vi "Do Request.vi"(7 "Controller Inputs":T2, 8 "error in (no error)":errorcluster, 11 "TestCSRFController in":refnum<class "TestCSRFController.lvclass">) -> (0 "error out":errorcluster, 5 "Controller Outputs":T1)   [LabVIEW 2020, in "TestCSRFController.lvclass"]
uses:
  TestCSRFController.lvclass
  HTTP Server/Controller Inputs.ctl
  HTTP Server/Arguments/Arguments.lvclass
  <vilib>/IlluminatedG/IG HTTP Utils/HTTP Utils/Request/Request.lvclass
  HTTP Server/Session/Session.lvclass
  HTTP Server/Controller Outputs.ctl
  <vilib>/IlluminatedG/IG HTTP Utils/HTTP Utils/Response/Response.lvclass
  TestCSRFController.lvclass/TestCSRFController.ctl
  <vilib>/IlluminatedG/IG HTTP Utils/HTTP Utils/FormField/FormField.lvclass
  HTTP Server/HTTP Server.lvlib
  <vilib>/IlluminatedG/lv-stream/URI/URI.lvclass
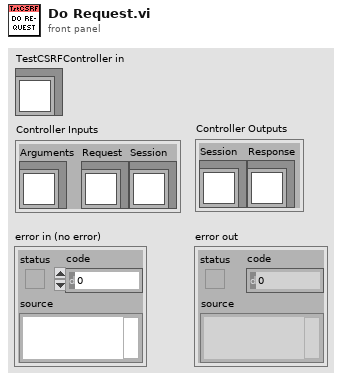
[diagram p1: front panel]
types:
  T1 = typedef "HTTP Server.lvlib/Controller Outputs.ctl" = cluster{"Session":refnum<class "Session.lvclass">, "Response":refnum<class "Response.lvclass">}
  T2 = typedef "HTTP Server.lvlib/Controller Inputs.ctl" = cluster{"Arguments":refnum<class "Arguments.lvclass">, "Request":refnum<class "Request.lvclass">, "Session":refnum<class "Session.lvclass">}
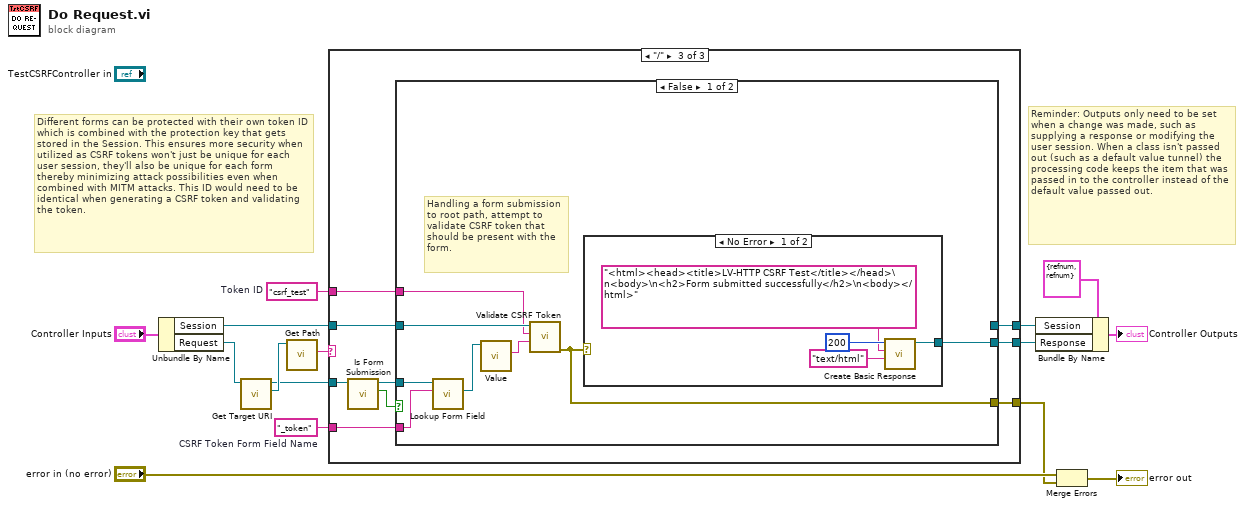
[diagram p0: block diagram]
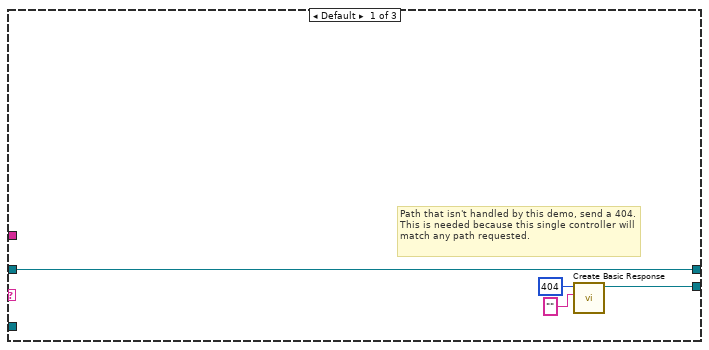
[diagram p2: hidden frame]
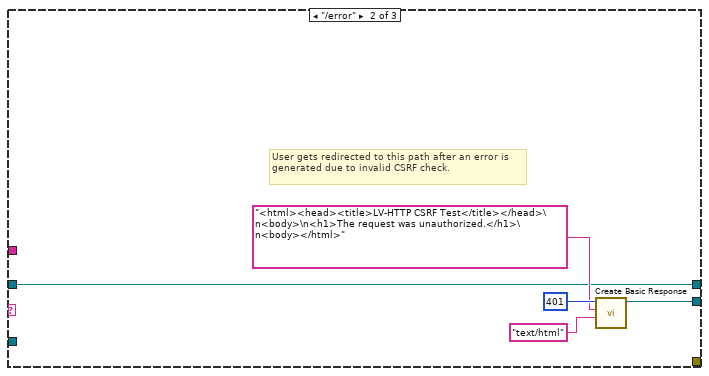
[diagram p3: hidden frame]
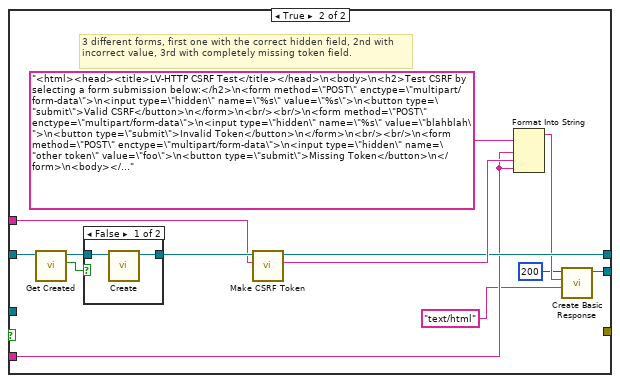
[diagram p5: hidden frame]
diagram:
  w11 = "_token"  # CSRF Token Form Field Name
  w12 = "csrf_test"  # Token ID
  # "Different forms can be protected with their own token ID which is combined with the protection key that gets stored in the Session. This ensures more security when utilized as CSRF tokens won't just be unique for each user session, they'll also be unique for each form thereby minimizing attack possibilities even when combined with MITM attacks. This ID would need to be identical when generating a CSRF token and validating the token."
  # "Reminder: Outputs only need to be set when a change was made, such as supplying a response or modifying the user session. When a class isn't passed out (such as a default value tunnel) the processing code keeps the item that was passed in to the controller instead of the default value passed out."
  n1 = Unbundle By Name("Controller Inputs") -> ("Session"=w13:refnum<class "Session.lvclass">, "Request"=w2:refnum<class "Request.lvclass">)
  n2 = call <vilib>:"Get Target URI.vi"("Request in"=w2) -> ("Target URI"=w7:refnum<class "URI.lvclass">, "Request out"=w5:refnum<class "Request.lvclass">)  [unwired: 8 in, 1 out]
  n3 = call <vilib>:"Get Path.vi"("URI in"=w7) -> ("Path"=w6:string)  [unwired: 8 in, 2 out]
  n4 = case shown="\"/\"" w6 {
    tunnel: w13 -> [w16 w21 w30]
    tunnel: w5 -> [_ _ w28]
    tunnel: [w17 w24 w33] -> w4
    tunnel: [w16 w21 w32] -> w3
    tunnel: w12 -> [_ _ w29]
    tunnel: w11 -> [_ _ w31]
    tunnel: [_ _ w25] -> w1
    frame Default {
      # "Path that isn't handled by this demo, send a 404. This is needed because this single controller will match any path requested."
      n5 = call <vilib>:"Create Basic Response.vi"("Payload"="", "Status Code"=u16 404) -> ("Response out"=w17:refnum<class "Response.lvclass">)  [unwired: 8 in, 1 out]
    }
    frame "/error" {
      # "User gets redirected to this path after an error is generated due to invalid CSRF check."
      n6 = call <vilib>:"Create Basic Response.vi"("Content-Type (text/plain)"="text/html", "Payload"="<html><head><title>LV-HTTP CSRF Test</title></head>\n<body>\n<h1>The request was unauthorized.</h1>\n<body></html>", "Status Code"=u16 401) -> ("Response out"=w24:refnum<class "Response.lvclass">)  [unwired: 7 in, 1 out]
    }
    frame "/" {
      n7 = call <vilib>:"Is Form Submission.vi"("Request in"=w28) -> ("Is Form Submission?"=w27:bool, "Request out"=w26:refnum<class "Request.lvclass">)  [unwired: 8 in, 1 out]
      n8 = case shown="False" w27 {
        tunnel: [w37 w58] -> w33
        tunnel: [_ w55] -> w32
        tunnel: w31 -> [w36 w54]
        tunnel: w30 -> [w39 w50]
        tunnel: w29 -> [w35 w46]
        tunnel: w26 -> [w38 _]
        tunnel: [w34 _] -> w25
        frame False {
          # "Handling a form submission to root path, attempt to validate CSRF token that should be present with the form."
          n9 = call <vilib>:"Lookup Form Field.vi"("Name"=w36, "Request in"=w38) -> ("Field"=w41:refnum<class "FormField.lvclass">)  [unwired: 6 in, 3 out]
          n10 = call <vilib>:"Value.vi"("FormField in"=w41) -> ("Value"=w40:string)  [unwired: 8 in, 2 out]
          n11 = call "Validate CSRF Token.vi"("Token"=w40, "Token ID"=w35, "Session In"=w39) -> ("error out"=w34:errorcluster)  [unwired: 7 in, 1 out]
          n12 = case shown="No Error" w34 {
            tunnel: [w45 _] -> w37
            frame No Error {
              n13 = call <vilib>:"Create Basic Response.vi"("Content-Type (text/plain)"="text/html", "Payload"="<html><head><title>LV-HTTP CSRF Test</title></head>\n<body>\n<h2>Form submitted successfully</h2>\n<body></html>", "Status Code"=u16 200) -> ("Response out"=w45:refnum<class "Response.lvclass">)  [unwired: 7 in, 1 out]
            }
            frame Error {
              # "Don't need to handle error here, we'll rely on passing the error out and the exception handling to generate a response."
            }
          }
        }
        frame True {
          # "3 different forms, first one with the correct hidden field, 2nd with incorrect value, 3rd with completely missing token field."
          n14 = call "Get Created.vi"("Session in"=w50) -> ("Created"=w49:bool, "Session out"=w48:refnum<class "Session.lvclass">)  [unwired: 8 in, 1 out]
          n15 = case shown="False" w49 {
            tunnel: w48 -> [w60 w61]
            tunnel: [w59 w61] -> w47
            frame False {
              n16 = call "Create.vi"("Session in"=w60) -> ("Session out"=w59:refnum<class "Session.lvclass">)  [unwired: 9 in, 1 out]
            }
            frame True {
            }
          }
          n17 = call "Make CSRF Token.vi"("Token ID"=w46, "Session In"=w47) -> ("Token"=w56:string, "Session"=w55:refnum<class "Session.lvclass">)  [unwired: 7 in, 1 out]
          n18 = Format Into String(format string="<html><head><title>LV-HTTP CSRF Test</title></head>\n<body>\n<h2>Test CSRF by selecting a form submission below:</h2>\n<form method=\"POST\" enctype=\"multipart/form-data\">\n<input type=\"hidden\" name=\"%s\" value=\"%s\">\n<button type=\"submit\">Valid CSRF</button>\n</form>\n<br/><br/>\n<form method=\"POST\" enctype=\"multipart/form-data\">\n<input type=\"hidden\" name=\"%s\" value=\"blahblah\">\n<button type=\"submit\">Invalid Token</button>\n</form>\n<br/><br/>\n<form method=\"POST\" enctype=\"multipart/form-data\">\n<input type=\"hidden\" name=\"other token\" value=\"foo\">\n<button type=\"submit\">Missing Token</button>\n</form>\n<body></html>", w54, w56, w54) -> (resulting string=w53:string)  [unwired: 2 in, 1 out]
          n19 = call <vilib>:"Create Basic Response.vi"("Content-Type (text/plain)"="text/html", "Payload"=w53, "Status Code"=u16 200) -> ("Response out"=w58:refnum<class "Response.lvclass">)  [unwired: 7 in, 1 out]
        }
      }
    }
  }
  n20 = Bundle By Name(cluster=T1 {"Session"=refnum, "Response"=refnum} ("Controller Outputs"), "Session"=w3, "Response"=w4) -> (→"Controller Outputs":T1)
  n21 = Merge Errors("error in (no error)", w1) -> (→"error out":errorcluster)
